vi "Rename File.vi"(8 "error in (no error)":errorcluster, 9 "Replace Subname":string="Template", 10 "New Subname":string, 11 "VI Path":path) -> (0 "error out":errorcluster)   [LabVIEW 2021, in "Plugin Generator.lvlib"]
uses:
  Plugin Generator.lvlib
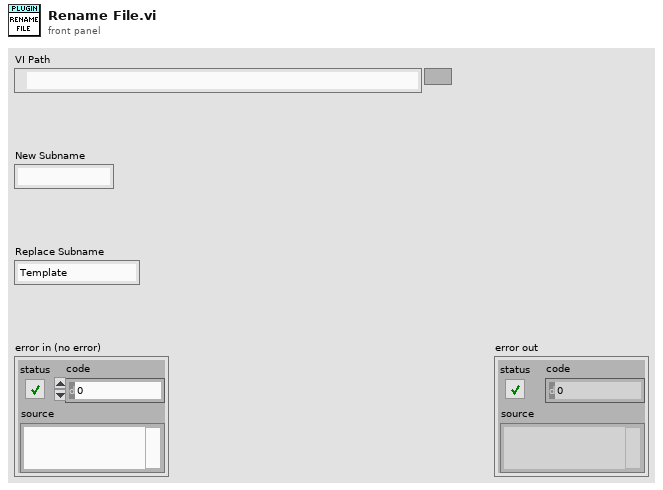
[diagram p1: front panel]
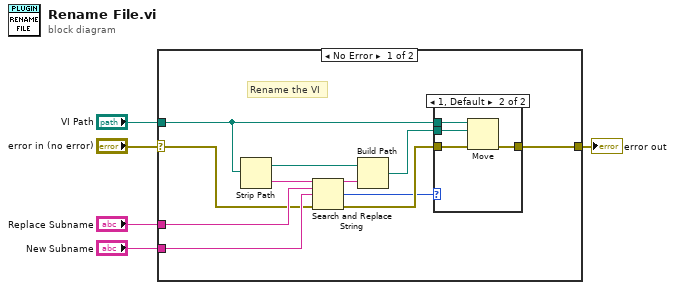
[diagram p0: block diagram]
diagram:
  n1 = case shown="No Error" "error in (no error)" {
    selector: "error in (no error)" -> [w12 w22]
    tunnel: [w16 w22] -> w1
    tunnel: "VI Path" -> [w13 _]
    tunnel: "New Subname" -> [w14 _]
    tunnel: "Replace Subname" -> [w15 _]
    frame No Error {
      # "Rename the VI"
      n2 = Strip Path(path=w13) -> (stripped path=w11:path, name=w8:string)
      n3 = Search and Replace String(input string=w8, search string=w15, replace string=w14, error in=w12) -> (result string=w7:string, number of replacements=w6:i32, error out=w9:errorcluster)  [unwired: 4 in, 1 out]
      n4 = Build Path(base path=w11, name or relative path=w7) -> (appended path=w10:path)
      n5 = case shown="1, Default" w6 {
        tunnel: w13 -> [_ w21]
        tunnel: w10 -> [_ w20]
        tunnel: [w17 w19] -> w16
        tunnel: w9 -> [w17 w18]
        frame 0 {
        }
        frame 1, Default {
          n6 = Move(source path=w21, error in=w18, 10:w20) -> (error out=w19:errorcluster)  [unwired: 2 in, 2 out]
        }
      }
    }
    frame Error {
    }
  }
  "error out" <- w1
